vi "Table-Get Visible Rows.vi"(0 "reference":refnum<vi>, 7 "Bounds":T1) -> (8 "Visible rows":i32)   [LabVIEW 2020]
uses:
  <vilib>/Utility/miscctls.llb/LVRectTypeDef.ctl
  <vilib>/Utility/miscctls.llb/LVRowAndColumnTypeDef.ctl
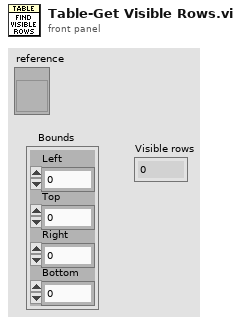
[diagram p1: front panel]
types:
  T1 = typedef "LVRectTypeDef.ctl" = cluster{"Left":i16, "Top":i16, "Right":i16, "Bottom":i16}
  T2 = typedef "LVRowAndColumnTypeDef.ctl" = cluster{"Row":i32, "Column":i32}
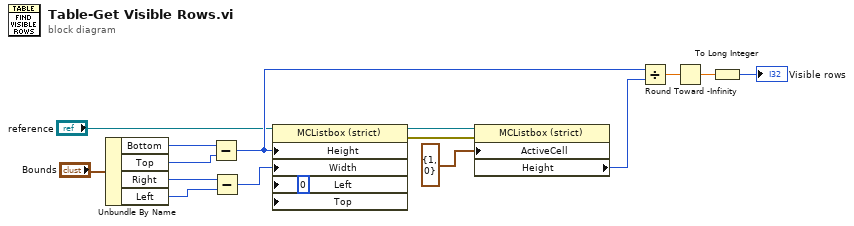
[diagram p0: block diagram]
diagram:
  w12 = 0 ("Position:Left")
  n1 = Unbundle By Name("Bounds") -> ("Bottom"=w5:i16, "Top"=w4:i16, "Right"=w3:i16, "Left"=w2:i16)
  n2 = Subtract(x=w5, y=w4) -> (x-y=w13:i16)
  n3 = Subtract(x=w3, y=w2) -> (x-y=w9:i16)
  n4 = property on="Property Node" class="MCListbox (strict)"(reference="reference", "Height"=w13, "Width"=w9, "Left"=w12, "Top"=w12) -> (reference out=w7:refnum<vi>, error out=w10:errorcluster)  [unwired: 1 in]
  n5 = property on="Property Node" class="MCListbox (strict)"(reference=w7, error in=w10, "ActiveCell"=T2 {"Row"=1, "Column"=0} ("Active Cell:Active Cell")) -> ("Height"=w14:u32)  [unwired: 2 out]
  n6 = Divide(x=w13, y=w14) -> (x/y=w15:dbl)
  n7 = Round Toward -Infinity(1:w15) -> (0:w16:dbl)
  n8 = To Long Integer(number=w16) -> (32bit integer=→"Visible rows":i32)
